vi "Fault View.vi"(10 "User Events in":refnum<class "User Events.lvclass">, 11 "M1M3 Support Events in":refnum<class "M1M3 Support Events.lvclass">) -> ()   [LabVIEW 2016]
uses:
  User Events/User Events.lvclass
  M1M3 Support Events/M1M3 Support Events.lvclass
  User Events/User Events.lvclass/User Events.ctl
  M1M3 Support Events/M1M3 Support Events.lvclass/M1M3 Support Events.ctl
  Typedefs/StateTypes.ctl
  <vilib>/Utility/error.llb/DialogType.ctl
  Typedefs/M1M3SupportEUI_TypeDefs.lvlib
panel:
  out "Fault":string
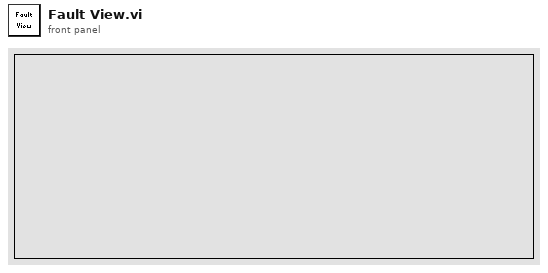
[diagram p1: front panel]
types:
  T1 = typedef "M1M3SupportEUI_TypeDefs.lvlib/M1M3 Support Events.ctl" = cluster{"M1M3 Support State":refnum<user-event>, "Inclinometer  Data":refnum<user-event>, "IMS Data":refnum<user-event>}
  T2 = typedef "M1M3SupportEUI_TypeDefs.lvlib/Publish Data Events.ctl" = cluster{"ErrorCode":refnum<user-event>}
  T3 = typedef "M1M3SupportEUI_TypeDefs.lvlib/StateTypes.ctl" = enum16{"Offline State", "Fault State", "Standby State", "Disabled State", "Enabled State", "Wait For User Input State", "Test Actuator State"}
  T4 = typedef "DialogType.ctl" = u16
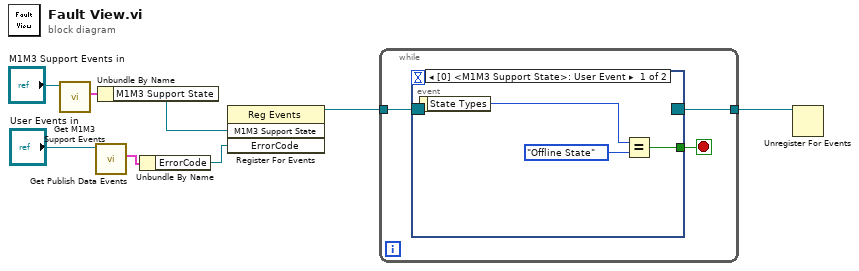
[diagram p0: block diagram]
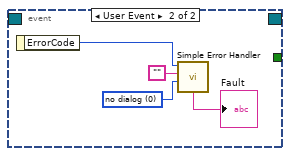
[diagram p2: hidden frame]
diagram:
  n1 = call "Get M1M3 Support Events.vi"("M1M3 Support Events in"="M1M3 Support Events in") -> ("M1M3 Support Events"=w6:T1)  [unwired: 9 in, 1 out]
  n2 = call "Get Publish Data Events.vi"("UserEvents in"="User Events in") -> ("Publish Data Events"=w8:T2)  [unwired: 9 in, 1 out]
  n3 = Unbundle By Name(w6) -> ("M1M3 Support State"=w4:refnum<user-event>)
  n4 = Unbundle By Name(w8) -> ("ErrorCode"=w3:refnum<user-event>)
  n5 = register-events(w4, w3) -> (reference out=w1:refnum<event-registration>)  [unwired: 2 in, 1 out]
  n6 = while {
    tunnel: w1 -> [w11]
    tunnel: [w10] -> w2
    stop <- w9 stop-if-true
    n7 = event shown="[0] <M1M3 Support State>: User Event" {
      selector: w11 -> [_ _]
      dyn-events: [_ _] -> w10
      timeout: _ -> [_ _]
      tunnel: [w13 _] -> w9
      event User Event {
        n8 = event-data() -> ("State Types"=w12:T3)  [unwired: 1 in]
        n9 = Equal?(x=w12, y=StateTypes."Offline State") -> (x = y?=w13:bool)
      }
      event User Event {
        w18 = T4 0 items=["no dialog", "OK message", "continue or stop message", "OK message + warnings", "continue/stop + warnings"] ("type of dialog (OK msg:1)")
        n10 = event-data() -> ("ErrorCode"=w16:i32)  [unwired: 1 in]
        n11 = call <vilib>:"Simple Error Handler.vi"("error code (no error:0)"=w16, "error source (\" \")"="", "type of dialog (OK msg:1)"=w18) -> ("message"=→"Fault":string)  [unwired: 2 in, 4 out]
      }
    }
  }
  n12 = Unregister For Events(event registration refnum=w2) -> ()  [unwired: 1 in, 1 out]
